vi "BRig_dataCurrent_T_generic.vi"() -> (2 "output_T_generic":i32)   [LabVIEW 2014]
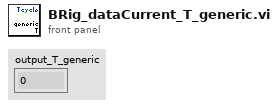
[diagram p1: front panel]
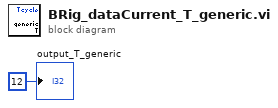
[diagram p0: block diagram]
diagram:
  "output_T_generic" <- 12 ("output_iBlock")
